vi "Parse 04 Puzzle.vi"(10 "Target Letters":string, 11 "Puzzle":string) -> (0 "Axcii Target Letters Out":u8[](array[numeric]), 2 "Letter Location Array Out":cluster{"Array":T1[]}[](array[cluster]), 3 "Ascii Byte Array Out":u8[][](array[numeric]))   [LabVIEW 2024]
uses:
  TypeDefs/Cluster Row-Column.ctl
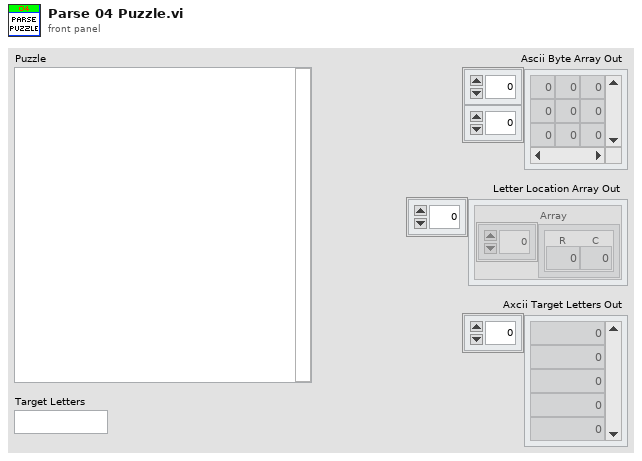
[diagram p1: front panel]
types:
  T1 = typedef "Cluster Row-Column.ctl" = cluster{"R":i32, "C":i32}
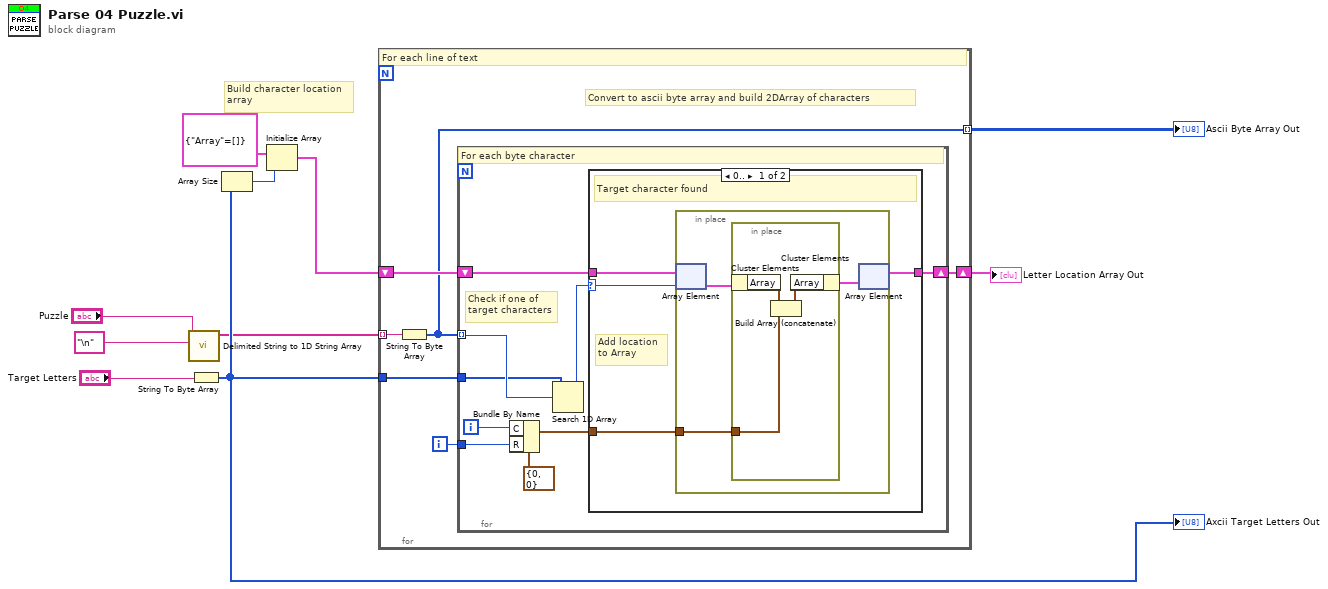
[diagram p0: block diagram]
diagram:
  # "Build character location\narray"
  n1 = call <vilib>:"Delimited String to 1D String Array.vi"("delimiter"="\n" ("delimiter (Tab)"), "delimited string"="Puzzle") -> ("string array"=w2:string[])  [unwired: 9 in]
  n2 = String To Byte Array(string="Target Letters") -> (unsigned byte array=w10:u8[])
  "Axcii Target Letters Out" <- w10
  n3 = Array Size(array=w10) -> (size(s)=w4:i32)
  n4 = Initialize Array(cluster{"Array":T1[]} {"Array"=[]}, w4) -> (w6:cluster{"Array":T1[]}[])
  n5 = for {
    tunnel: w2 -> [w16] mode=indexing
    tunnel: w10 -> [w14]
    shift-right: [w12] -> w7
    shift-left: w6 -> [w13]
    tunnel: [w11] -> w8 mode=indexing
    i -> [w15]
    # "Convert to ascii byte array and build 2DArray of characters"
    # "For each line of text"
    n6 = String To Byte Array(string=w16) -> (unsigned byte array=w11:u8[])
    n7 = for {
      tunnel: w11 -> [w25] mode=indexing
      tunnel: w15 -> [w18]
      tunnel: w14 -> [w21]
      shift-right: [w22] -> w12
      shift-left: w13 -> [w23]
      i -> [w19]
      # "Check if one of\ntarget characters"
      # "For each byte character"
      n8 = Bundle By Name(cluster=T1 {"R"=0, "C"=0}, "C"=w19, "R"=w18) -> (w17:T1)
      n9 = Search 1D Array(1D array=w21, element=w25) -> (index of element=w24:i32)  [unwired: 1 in]
      n10 = case shown="0.." w24 {
        selector: w24 -> [w26 _]
        tunnel: w17 -> [w29 _]
        tunnel: w23 -> [w28 w36]
        tunnel: [w27 w36] -> w22
        frame 0.. {
          # "Add location\nto Array"
          # "Target character found"
          n11 = in-place {
            in-place-border: w29 -> [w31]
            n12 = in-place-array #1(w28, w26) -> (w32:cluster{"Array":T1[]})
            n13 = in-place {
              in-place-border: w31 -> [w34]
              n14 = in-place-cluster #2(w32) -> ("Array"=w35:T1[])
              n15 = Build Array (concatenate)(w35, w34) -> (w33:T1[])
              n16 = in-place-cluster #2("Array"=w33) -> (w30:cluster{"Array":T1[]})
            }
            n17 = in-place-array #1(w30) -> (w27:cluster{"Array":T1[]}[])  [unwired: 1 out]
          }
        }
        frame ..-1 {
          # "target character not found"
        }
      }
    }
  }
  "Ascii Byte Array Out" <- w8
  "Letter Location Array Out" <- w7
